vi "例2_连续运动.vi"() -> ()   [LabVIEW 2012]
panel:
  in  "软件复位":bool
  in  "硬件复位":bool
  in  "总线状态":string
  in  "轴状态机":string
  in  "退出程序":bool
  in  "卡号":dbl
  in  "运动方向":enum32{"负方向", "正方向"}(radio)
  in  "指令清零":bool
  in  "设置脉冲当量":bool
  in  "停止运动":bool
  in  "执行运动":bool
  in  "反馈位置 unit":dbl
  in  "当前位置 unit":dbl
  in  "当前速度 unit/s":dbl
  in  "运动状态":string
  in  "在线变速":bool
  in  "变速时间 s":dbl
  in  "变速的运行速度 unit/s":dbl
  in  "停止速度 unit/s":dbl
  in  "S段时间 s":dbl
  in  "减速时间 s":dbl
  in  "加速时间 s":dbl
  in  "运行速度 unit/s":dbl
  in  "起始速度 unit/s":dbl
  in  "脉冲当量  pulse/unit":dbl
  in  "电机轴号":dbl
  # "输入参数"
  # "在线变速"
  # "信息显示"
  # "运动方向"
  # "复位"
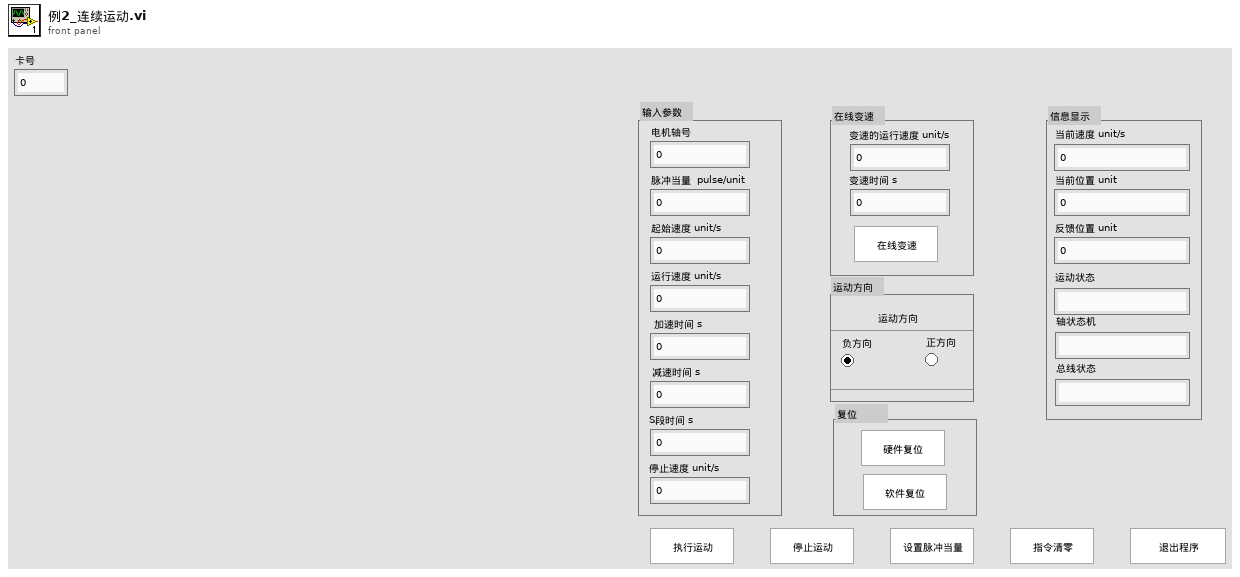
[diagram p1: front panel]
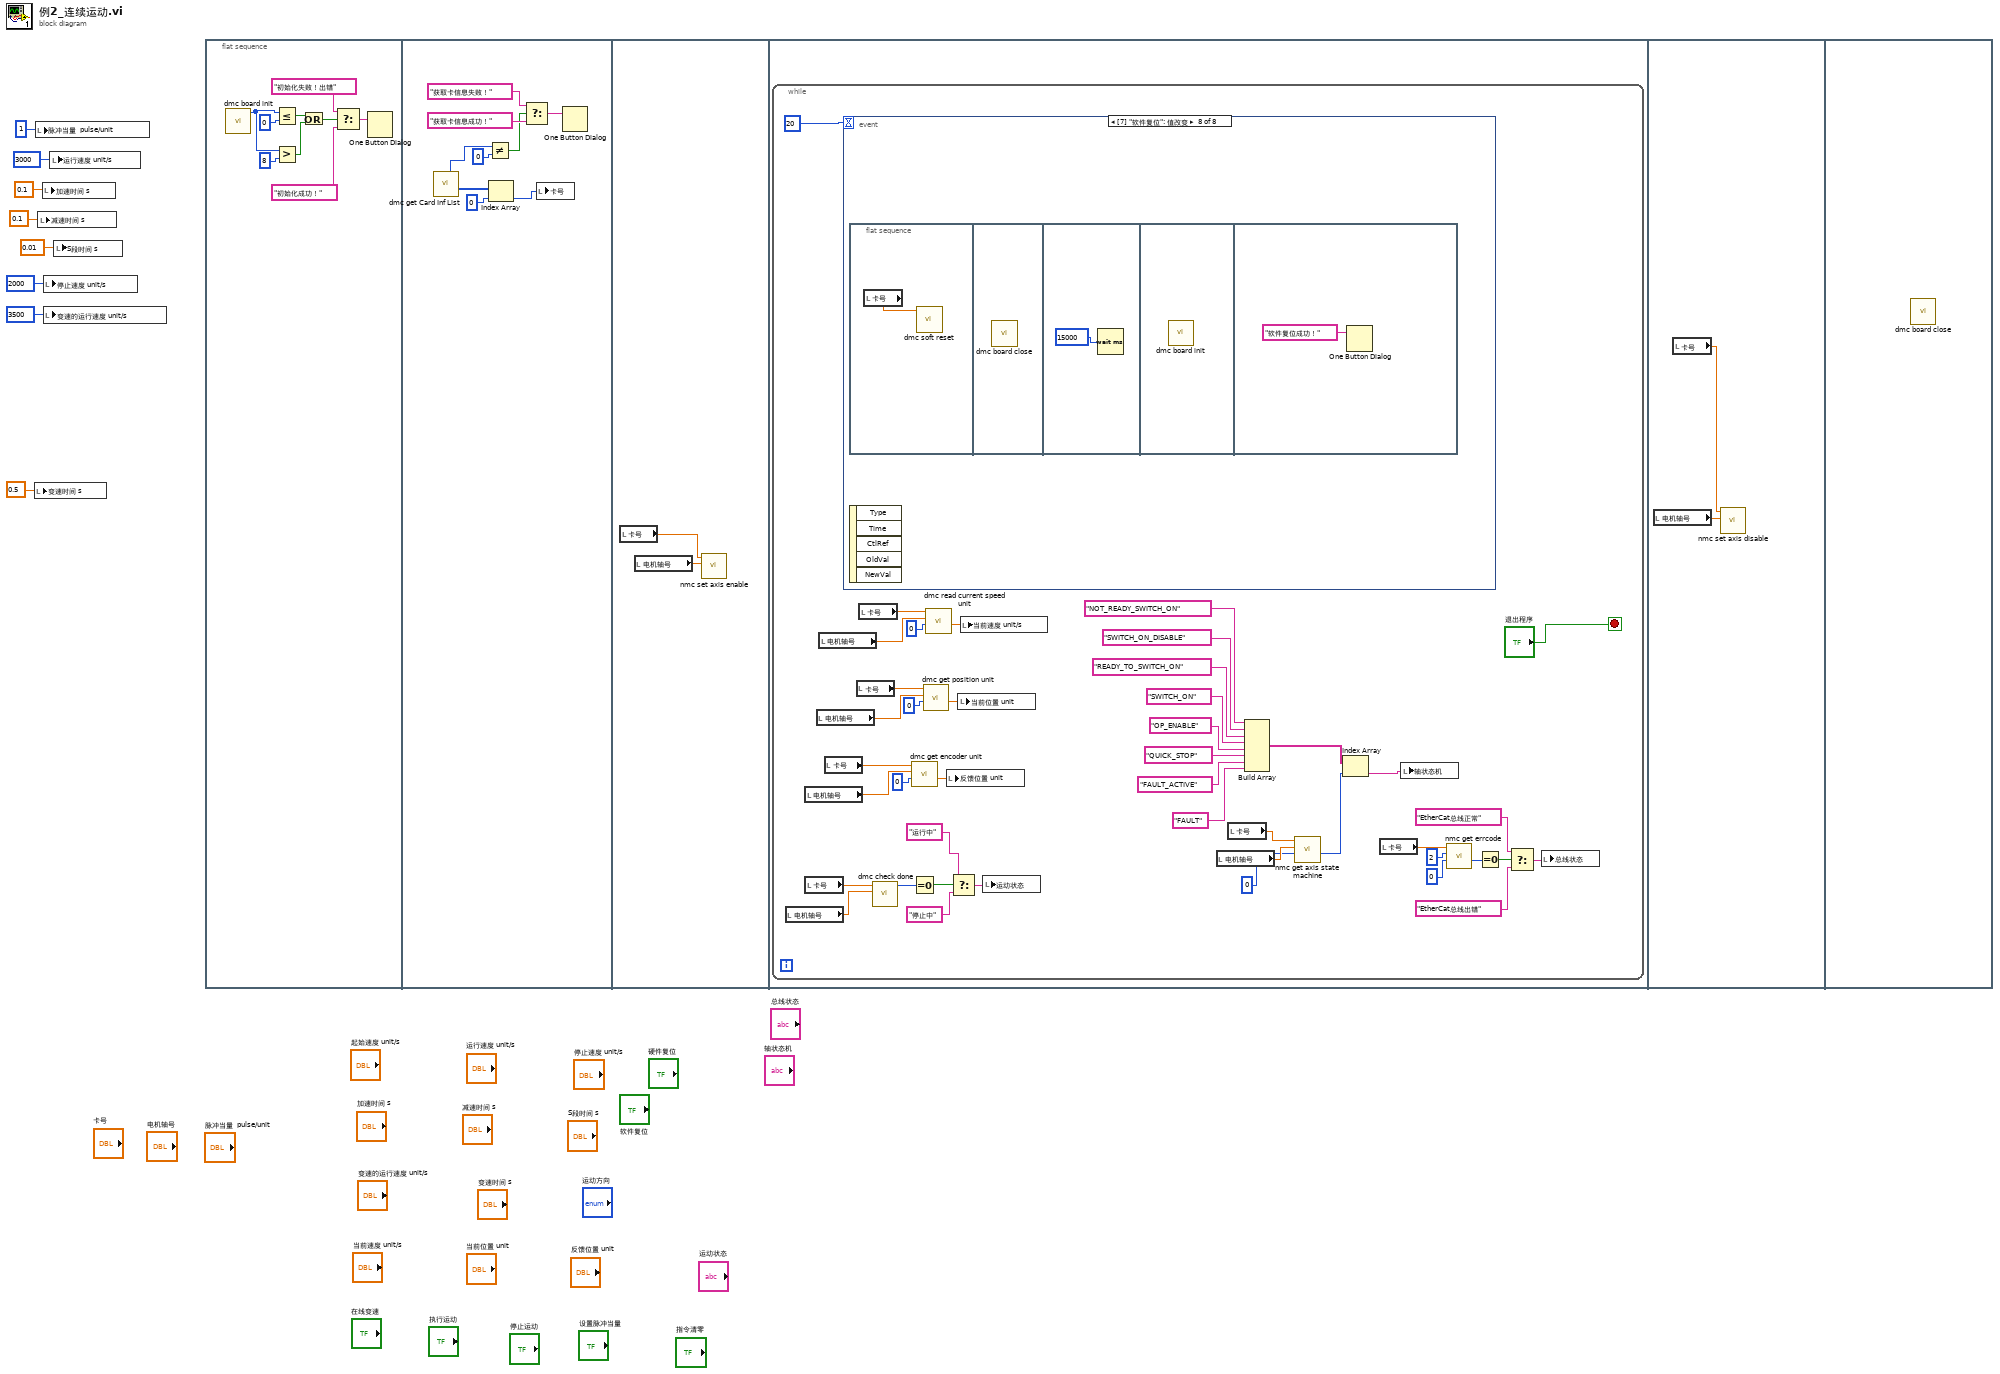
[diagram p0: block diagram]
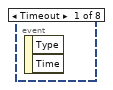
[diagram p2: hidden frame]
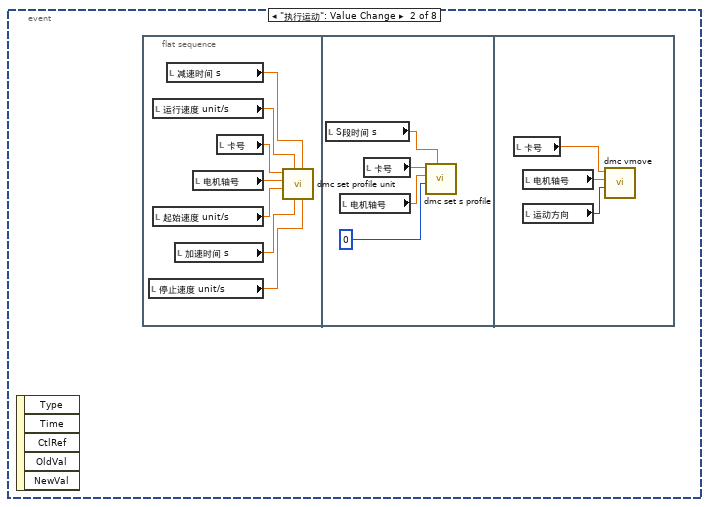
[diagram p3: hidden frame]
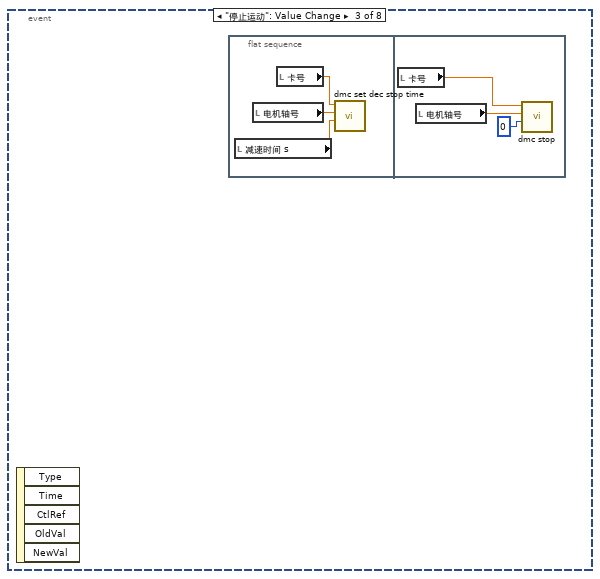
[diagram p4: hidden frame]
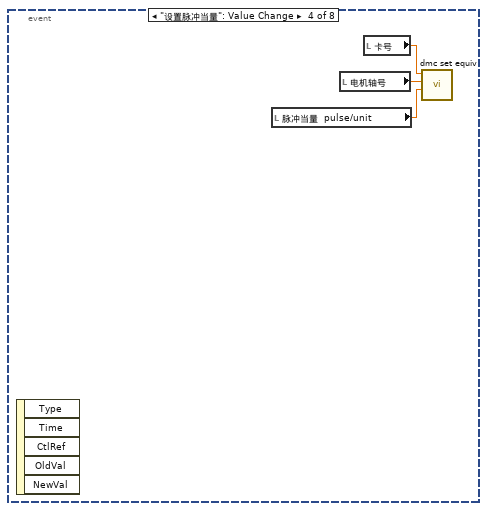
[diagram p5: hidden frame]
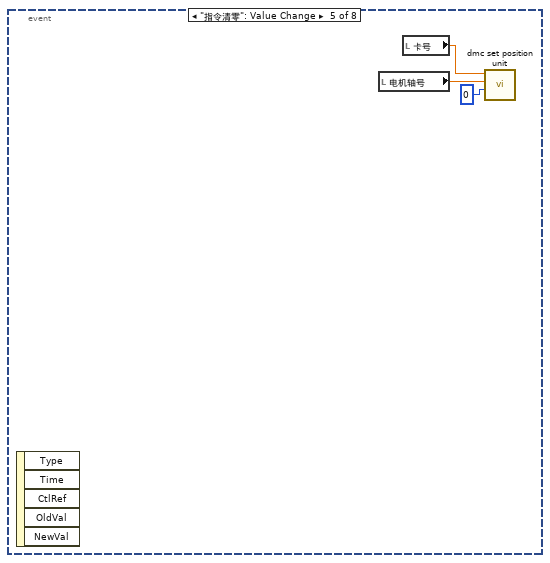
[diagram p6: hidden frame]
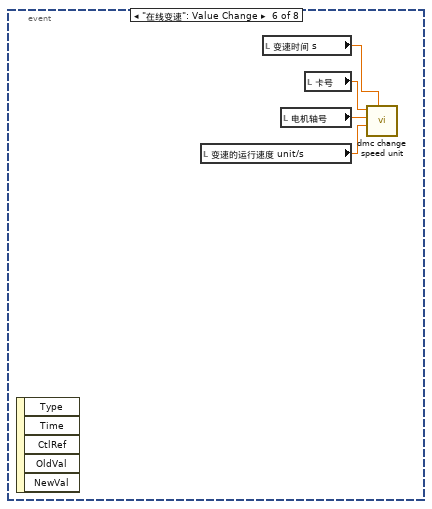
[diagram p7: hidden frame]
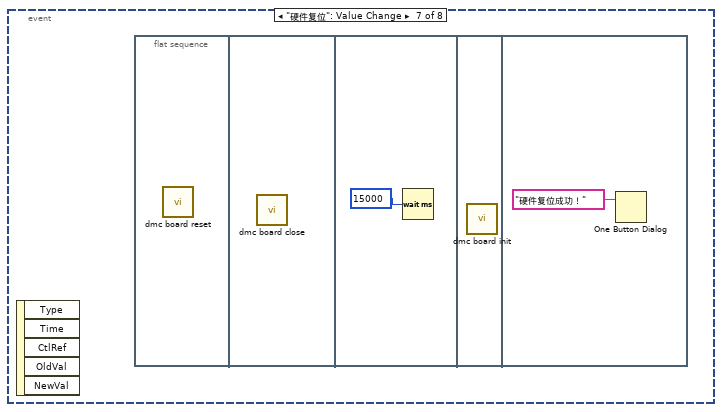
[diagram p8: hidden frame]
diagram:
  n1 = local write "变速时间 s"(0.5) -> ()
  n2 = local write "脉冲当量  pulse/unit"(1) -> ()
  n3 = local write "减速时间 s"(0.1) -> ()
  n4 = local write "加速时间 s"(0.1) -> ()
  n5 = local write "停止速度 unit/s"(2000) -> ()
  n6 = local write "变速的运行速度 unit/s"(3500) -> ()
  n7 = local write "运行速度 unit/s"(3000) -> ()
  n8 = local write "S段时间 s"(0.01) -> ()
  n9 = flat-sequence {
    frame #0 {
      n10 = call "dmc board init.vi"() -> ("function return"=w10:i16)  [unwired: 10 in, 1 out]
      n11 = Less Or Equal?(x=w10, y=0) -> (x <= y?=w13:bool)
      n12 = Greater?(x=w10, y=8) -> (0:w12:bool)
      n13 = Or(x=w13, y=w12) -> (x .or. y?=w14:bool)
      n14 = Select(t="初始化失败！出错", s=w14, f="初始化成功！") -> (s? t:f=w16:string)
      n15 = One Button Dialog(message=w16) -> ()  [unwired: 1 in, 1 out]
    }
    frame #1 {
      n16 = call "dmc get Card Inf List.vi"() -> ("CardIdList out"=w20:u16[], "function return"=w21:i16)  [unwired: 7 in, 3 out]
      n17 = Not Equal?(x=w21, y=0) -> (x != y?=w23:bool)
      n18 = Index Array(array=w20, index=0) -> (element=w18:u16)
      n19 = Select(t="获取卡信息失败！", s=w23, f="获取卡信息成功！") -> (s? t:f=w26:string)
      n20 = local write "卡号"(w18) -> ()
      n21 = One Button Dialog(message=w26) -> ()  [unwired: 1 in, 1 out]
    }
    frame #2 {
      n22 = local read "卡号"() -> (w28:dbl)
      n23 = local read "电机轴号"() -> (w27:dbl)
      n24 = call "nmc set axis enable.vi"("axis"=w27, "CardNo"=w28) -> ()  [unwired: 8 in, 2 out]
    }
    frame #3 {
      n25 = while {
        stop <- "退出程序" stop-if-true
        n26 = local read "电机轴号"() -> (w53:dbl)
        n27 = local read "电机轴号"() -> (w61:dbl)
        n28 = local read "卡号"() -> (w54:dbl)
        n29 = local read "电机轴号"() -> (w65:dbl)
        n30 = local read "电机轴号"() -> (w69:dbl)
        n31 = local read "卡号"() -> (w62:dbl)
        n32 = event shown="[7] \"软件复位\": 值改变" {
          selector: _ -> [_ _ _ _ _ _ _ _]
          dyn-events: _ -> [_ _ _ _ _ _ _ _]
          timeout: 20 -> [_ _ _ _ _ _ _ _]
          event Timeout {
            n33 = event-data() -> ()  [unwired: 1 in, 2 out]
          }
          event "执行运动": Value Change {
            n34 = event-data() -> ()  [unwired: 1 in, 5 out]
            n35 = flat-sequence {
              frame #0 {
                n36 = local read "停止速度 unit/s"() -> (w74:dbl)
                n37 = local read "运行速度 unit/s"() -> (w73:dbl)
                n38 = local read "起始速度 unit/s"() -> (w76:dbl)
                n39 = local read "减速时间 s"() -> (w72:dbl)
                n40 = local read "加速时间 s"() -> (w75:dbl)
                n41 = local read "电机轴号"() -> (w77:dbl)
                n42 = local read "卡号"() -> (w78:dbl)
                n43 = call "dmc set profile unit.vi"("Stop_Vel"=w74, "Tdec"=w72, "Tacc"=w75, "Max_Vel"=w73, "Min_Vel"=w76, "axis"=w77, "CardNo"=w78) -> ()  [unwired: 3 in, 2 out]
              }
              frame #1 {
                n44 = local read "S段时间 s"() -> (w79:dbl)
                n45 = local read "电机轴号"() -> (w81:dbl)
                n46 = local read "卡号"() -> (w82:dbl)
                n47 = call "dmc set s profile.vi"("s_para"=w79, "s_mode"=0, "axis"=w81, "CardNo"=w82) -> ()  [unwired: 6 in, 2 out]
              }
              frame #2 {
                n48 = local read "卡号"() -> (w85:dbl)
                n49 = local read "电机轴号"() -> (w84:dbl)
                n50 = local read "运动方向"() -> (w83:enum32{"负方向", "正方向"})
                n51 = call "dmc vmove.vi"("dir"=w83, "axis"=w84, "CardNo"=w85) -> ()  [unwired: 7 in, 2 out]
              }
            }
          }
          event "停止运动": Value Change {
            n52 = event-data() -> ()  [unwired: 1 in, 5 out]
            n53 = flat-sequence {
              frame #0 {
                n54 = local read "减速时间 s"() -> (w88:dbl)
                n55 = local read "电机轴号"() -> (w87:dbl)
                n56 = local read "卡号"() -> (w86:dbl)
                n57 = call "dmc set dec stop time.vi"("time"=w88, "axis"=w87, "CardNo"=w86) -> ()  [unwired: 7 in, 2 out]
              }
              frame #1 {
                n58 = local read "卡号"() -> (w89:dbl)
                n59 = local read "电机轴号"() -> (w91:dbl)
                n60 = call "dmc stop.vi"("stop_mode"=0, "axis"=w91, "CardNo"=w89) -> ()  [unwired: 7 in, 2 out]
              }
            }
          }
          event "设置脉冲当量": Value Change {
            n61 = event-data() -> ()  [unwired: 1 in, 5 out]
            n62 = local read "脉冲当量  pulse/unit"() -> (w93:dbl)
            n63 = local read "电机轴号"() -> (w94:dbl)
            n64 = local read "卡号"() -> (w92:dbl)
            n65 = call "dmc set equiv.vi"("equiv"=w93, "axis"=w94, "CardNo"=w92) -> ()  [unwired: 7 in, 2 out]
          }
          event "指令清零": Value Change {
            n66 = event-data() -> ()  [unwired: 1 in, 5 out]
            n67 = local read "电机轴号"() -> (w97:dbl)
            n68 = local read "卡号"() -> (w95:dbl)
            n69 = call "dmc set position unit.vi"("pos"=0, "axis"=w97, "CardNo"=w95) -> ()  [unwired: 7 in, 2 out]
          }
          event "在线变速": Value Change {
            n70 = event-data() -> ()  [unwired: 1 in, 5 out]
            n71 = local read "变速的运行速度 unit/s"() -> (w100:dbl)
            n72 = local read "变速时间 s"() -> (w99:dbl)
            n73 = local read "电机轴号"() -> (w101:dbl)
            n74 = local read "卡号"() -> (w98:dbl)
            n75 = call "dmc change speed unit.vi"("Taccdec"=w99, "New_Vel"=w100, "axis"=w101, "CardNo"=w98) -> ()  [unwired: 6 in, 2 out]
          }
          event "硬件复位": Value Change {
            n76 = event-data() -> ()  [unwired: 1 in, 5 out]
            n77 = flat-sequence {
              frame #0 {
                n78 = call "dmc board reset.vi"() -> ()  [unwired: 10 in, 2 out]
              }
              frame #1 {
                n79 = call "dmc board close.vi"() -> ()  [unwired: 10 in, 2 out]
              }
              frame #2 {
                n80 = Wait (ms)(milliseconds to wait=15000) -> ()  [unwired: 1 out]
              }
              frame #3 {
                n81 = call "dmc board init.vi"() -> ()  [unwired: 10 in, 2 out]
              }
              frame #4 {
                n82 = One Button Dialog(message="硬件复位成功！") -> ()  [unwired: 1 in, 1 out]
              }
            }
          }
          event "软件复位": Value Change {
            n83 = flat-sequence {
              frame #0 {
                n84 = local read "卡号"() -> (w104:dbl)
                n85 = call "dmc soft reset.vi"("CardNo"=w104) -> ()  [unwired: 9 in, 2 out]
              }
              frame #1 {
                n86 = call "dmc board close.vi"() -> ()  [unwired: 10 in, 2 out]
              }
              frame #2 {
                n87 = Wait (ms)(milliseconds to wait=15000) -> ()  [unwired: 1 out]
              }
              frame #3 {
                n88 = call "dmc board init.vi"() -> ()  [unwired: 10 in, 2 out]
              }
              frame #4 {
                n89 = One Button Dialog(message="软件复位成功！") -> ()  [unwired: 1 in, 1 out]
              }
            }
            n90 = event-data() -> ()  [unwired: 1 in, 5 out]
          }
        }
        n91 = local read "卡号"() -> (w66:dbl)
        n92 = local read "卡号"() -> (w70:dbl)
        n93 = call "dmc check done.vi"("axis"=w53, "CardNo"=w54) -> ("function return"=w55:i16)  [unwired: 8 in, 1 out]
        n94 = call "dmc get encoder unit.vi"("pos"=0, "axis"=w61, "CardNo"=w62) -> ("pos out"=w59:dbl)  [unwired: 6 in, 2 out]
        n95 = Equal To 0?(x=w55) -> (x = 0?=w58:bool)
        n96 = call "dmc get position unit.vi"("pos"=0, "axis"=w65, "CardNo"=w66) -> ("pos out"=w63:dbl)  [unwired: 6 in, 2 out]
        n97 = call "dmc read current speed unit.vi"("current_speed"=0, "axis"=w69, "CardNo"=w70) -> ("current_speed out"=w67:dbl)  [unwired: 6 in, 2 out]
        n98 = local write "反馈位置 unit"(w59) -> ()
        n99 = Select(t="运行中" ("当前状态"), s=w58, f="停止中" ("当前状态")) -> (s? t:f=w52:string)
        n100 = local write "当前位置 unit"(w63) -> ()
        n101 = local write "当前速度 unit/s"(w67) -> ()
        n102 = local write "运动状态"(w52) -> ()
        n103 = local read "电机轴号"() -> (w40:dbl)
        n104 = local read "卡号"() -> (w41:dbl)
        n105 = Build Array("NOT_READY_SWITCH_ON", "SWITCH_ON_DISABLE", "READY_TO_SWITCH_ON", "SWITCH_ON", "OP_ENABLE", "QUICK_STOP", "FAULT_ACTIVE", "FAULT") -> (w43:string[])
        n106 = call "nmc get axis state machine.vi"("Axis_StateMachine"=0, "axis"=w40, "CardNo"=w41) -> ("Axis_StateMachine out"=w38:u16)  [unwired: 6 in, 2 out]
        n107 = Index Array(array=w43, index=w38) -> (element=w37:string)
        n108 = local read "卡号"() -> (w29:dbl)
        n109 = local write "轴状态机"(w37) -> ()
        n110 = call "nmc get errcode.vi"("Errcode"=0, "channel"=2, "CardNo"=w29) -> ("Errcode out"=w35:u16)  [unwired: 6 in, 2 out]
        n111 = Equal To 0?(x=w35) -> (x = 0?=w34:bool)
        n112 = Select(t="EtherCat总线正常" ("当前状态"), s=w34, f="EtherCat总线出错" ("当前状态")) -> (s? t:f=w31:string)
        n113 = local write "总线状态"(w31) -> ()
      }
    }
    frame #4 {
      n114 = local read "电机轴号"() -> (w107:dbl)
      n115 = local read "卡号"() -> (w108:dbl)
      n116 = call "nmc set axis disable.vi"("axis"=w107, "CardNo"=w108) -> ()  [unwired: 8 in, 2 out]
    }
    frame #5 {
      n117 = call "dmc board close.vi"() -> ()  [unwired: 10 in, 2 out]
    }
  }
